vi "TSET_6517.vi"(3 "Address No.":i8=2, 8 "T-Ending, C":dbl=300.0, 9 "VISA resource name":refnum<visa-resource-name> caption="VISA资源名称", 10 "cooling/heating rate, C/min":dbl=10.0) -> ()   [LabVIEW 2017]
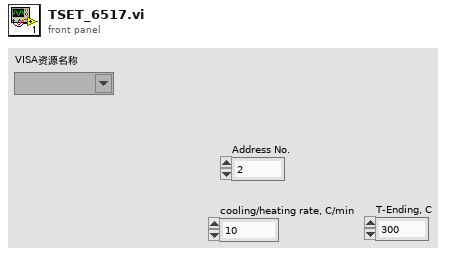
[diagram p1: front panel]
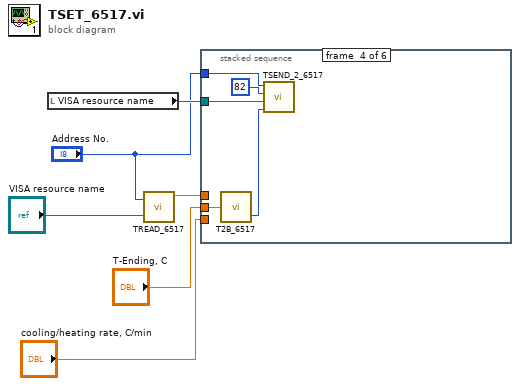
[diagram p0: block diagram]
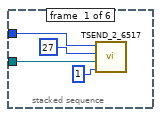
[diagram p2: hidden frame]
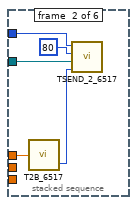
[diagram p3: hidden frame]
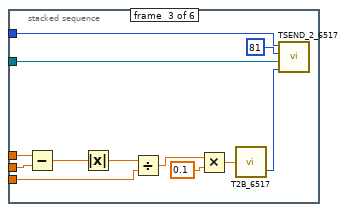
[diagram p4: hidden frame]
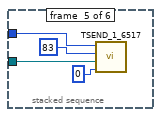
[diagram p5: hidden frame]
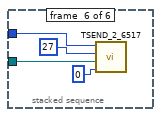
[diagram p6: hidden frame]
diagram:
  n1 = local read "VISA resource name"() -> (w5:refnum<visa-resource-name>)
  n2 = call "TREAD_6517.vi"("Address No."="Address No.", "VISA resource name"="VISA resource name") -> ("PV"=w4:dbl)  [unwired: 3 out]
  n3 = stacked-sequence {
    tunnel: "Address No." -> [w10 w15 w19 w31 w35 w40]
    tunnel: w4 -> [_ w12 w27 _ _ _]
    tunnel: "T-Ending, C" -> [_ _ w26 w32 _ _]
    tunnel: "cooling/heating rate, C/min" -> [_ _ w23 _ _ _]
    tunnel: w5 -> [w7 w11 w18 w30 w33 w38]
    frame #0 {
      n4 = call "TSEND_2_6517.vi"("SettingValue"=1, "VISA resource name"=w7, "No. for reading (Dec.)"=27, "Address No."=w10) -> ()  [unwired: 2 out]
    }
    frame #1 {
      n5 = call "T2B_6517.vi"("Temperature"=w12) -> ("16Bit(2Byte) value"=w13:u16)  [unwired: 1 out]
      n6 = call "TSEND_2_6517.vi"("SettingValue"=w13, "VISA resource name"=w11, "No. for reading (Dec.)"=80, "Address No."=w15) -> ()  [unwired: 2 out]
    }
    frame #2 {
      n7 = Subtract(x=w27, y=w26) -> (x-y=w25:dbl)
      n8 = Absolute Value(x=w25) -> (abs(x)=w24:dbl)
      n9 = Divide(x=w24, y=w23) -> (x/y=w22:dbl)
      n10 = Multiply(x=w22, y=0.1) -> (x*y=w20:dbl)
      n11 = call "T2B_6517.vi"("Temperature"=w20) -> ("16Bit(2Byte) value"=w16:u16)  [unwired: 1 out]
      n12 = call "TSEND_2_6517.vi"("SettingValue"=w16, "VISA resource name"=w18, "No. for reading (Dec.)"=81, "Address No."=w19) -> ()  [unwired: 2 out]
    }
    frame #3 {
      n13 = call "T2B_6517.vi"("Temperature"=w32) -> ("16Bit(2Byte) value"=w28:u16)  [unwired: 1 out]
      n14 = call "TSEND_2_6517.vi"("SettingValue"=w28, "VISA resource name"=w30, "No. for reading (Dec.)"=82, "Address No."=w31) -> ()  [unwired: 2 out]
    }
    frame #4 {
      n15 = call "TSEND_1_6517.vi"("SettingValue"=0, "VISA resource name"=w33, "No. for reading (Dec.)"=83, "Address No."=w35) -> ()  [unwired: 2 out]
    }
    frame #5 {
      n16 = call "TSEND_2_6517.vi"("SettingValue"=0, "VISA resource name"=w38, "No. for reading (Dec.)"=27, "Address No."=w40) -> ()  [unwired: 2 out]
    }
  }
